vi "determine_positive_channel.vi"(8 "error in (no error)":errorcluster, 11 "UI in":T1) -> (0 "error out":errorcluster, 2 "determined_channels":T5, 3 "UI out":T1)   [LabVIEW 2017]
uses:
  classes/dc_power_supply/DC_power_supply.lvclass
  <instrlib>/PICOTEST M352XA/Public/Controls/Function.ctl
  types/channels_enum.ctl
  types/motech_set_value_cluster.ctl
  ui_buttons.ctl
  types/boc_type.ctl
  ui.ctl
  classes/report/Report.lvclass
panel:
  in  "motech_set_value":T6={"voltage"=0.0, "current"=0.01, "channel"=enum."1"}
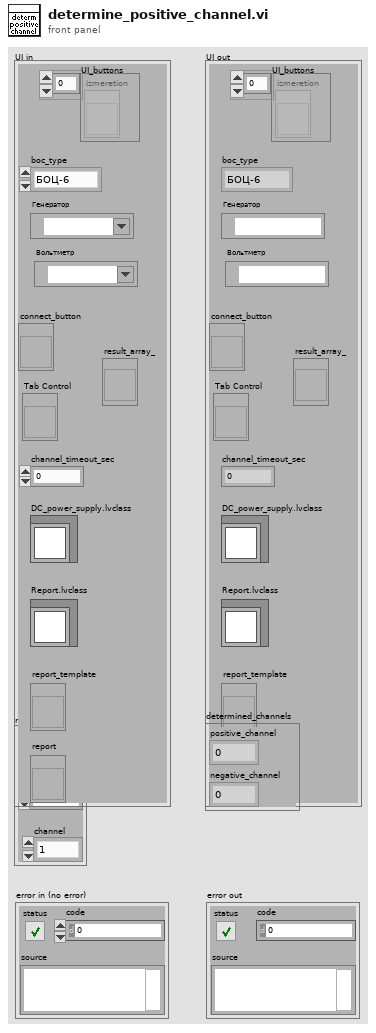
[diagram p1: front panel]
types:
  T1 = typedef "ui.ctl" = cluster{"UI_buttons":T2, "Tab Control":refnum<vi>, "connect_button":refnum<vi>, "generator":refnum<visa-resource-name>, "voltmetr":refnum<visa-resource-name>, "channel_timeout_sec":dbl, "boc_type":T3, "result_array_":refnum<vi>, "DC_power_supply.lvclass":refnum<class "DC_power_supply.lvclass">, "Report.lvclass":refnum<class "Report.lvclass">, "report_template":refnum<vi>, "report":refnum<vi>}
  T2 = typedef "ui_buttons.ctl" = refnum<vi>[]
  T3 = typedef "boc_type.ctl" = enum16{"БОЦ-6", "БОЦ-12"}
  T4 = typedef "channels_enum.ctl" = enum16{"0", "1", "2"}
  T5 = cluster{"positive_channel":T4, "negative_channel":T4}
  T6 = typedef "motech_set_value_cluster.ctl" = cluster{"voltage":dbl, "current":dbl, "channel":T4}
  T7 = typedef "Function.ctl" = enum16{"VOLTage:DC", "VOLTage:DC:RATio", "VOLTage:AC", "CURRent:DC", "CURRent:AC", "RESistance", "FRESistance", "FREQuency", "PERiod", "FREQuency:CURRent", "PERiod:CURRent", "CAPacitance", "CONTinuity", "DIODe", "TCOuple", "TEMPerature"}
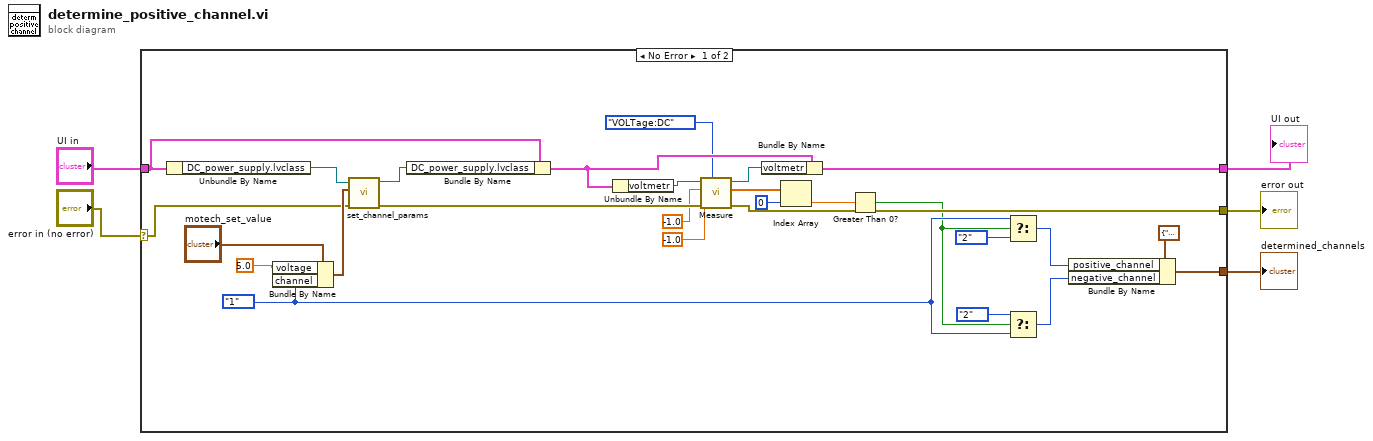
[diagram p0: block diagram]
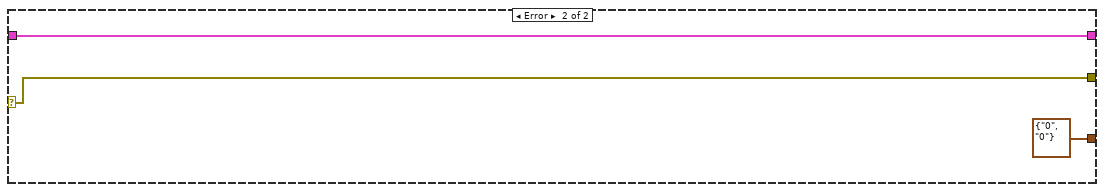
[diagram p2: hidden frame]
diagram:
  n1 = case shown="No Error" "error in (no error)" {
    selector: "error in (no error)" -> [w6 w34]
    tunnel: [w32 w35] -> w5
    tunnel: [w29 T5 {"positive_channel"=enum."0", "negative_channel"=enum."0"}] -> w4
    tunnel: [w28 w34] -> w3
    tunnel: "UI in" -> [w9 w35]
    frame No Error {
      w24 = channels_enum."1" ("channel")
      n2 = Unbundle By Name(w9) -> ("DC_power_supply.lvclass"=w7:refnum<class "DC_power_supply.lvclass">)
      n3 = Bundle By Name(cluster="motech_set_value", "voltage"=5.0, "channel"=w24) -> (w16:T6)
      n4 = call-dynamic "set_channel_params.vi"("error in (no error)"=w6, "motech_set_value"=w16, "DC_power_supply in"=w7) -> ("error out"=w14:errorcluster, "DC_power_supply out"=w8:refnum<class "DC_power_supply.lvclass">)  [unwired: 7 in]
      n5 = Bundle By Name(cluster=w9, "DC_power_supply.lvclass"=w8) -> (w30:T1)
      n6 = Unbundle By Name(w30) -> ("voltmetr"=w12:refnum<visa-resource-name>)
      n7 = call <instrlib>:"Measure.vi"("Function"=Function."VOLTage:DC", "error in (no error)"=w14, "Resolution"=-1.0, "Range"=-1.0, "VISA resource name"=w12) -> ("error out"=w28:errorcluster, "Measurements"=w18:dbl[], "VISA resource name out"=w31:refnum<visa-resource-name>)  [unwired: 4 in]
      n8 = Bundle By Name(cluster=w30, "voltmetr"=w31) -> (w32:T1)
      n9 = Index Array(array=w18, index=0) -> (element=w19:dbl)
      n10 = Greater Than 0?(x=w19) -> (x > 0?=w22:bool)
      n11 = Select(t=w24, s=w22, f=channels_enum."2") -> (s? t:f=w21:T4)
      n12 = Select(t=channels_enum."2" ("f"), s=w22, f=w24) -> (s? t:f=w25:T4)
      n13 = Bundle By Name(cluster=T5 {"positive_channel"=enum."2", "negative_channel"=enum."2"}, "positive_channel"=w21, "negative_channel"=w25) -> (w29:T5)
    }
    frame Error {
    }
  }
  "UI out" <- w5
  "determined_channels" <- w4
  "error out" <- w3
